vi "Handle Response.vi"(7 "Processing In":refnum<class "Processing.lvclass">, 11 "Response Handler in":refnum<class "Response Handler.lvclass">) -> (0 "error out":errorcluster, 5 "Processing":refnum<class "Processing.lvclass">)   [LabVIEW 2020, in "HTTP Server.lvlib" / "Response Handler.lvclass"]
uses:
  Response Handler.lvclass
  Processing/Processing.lvclass
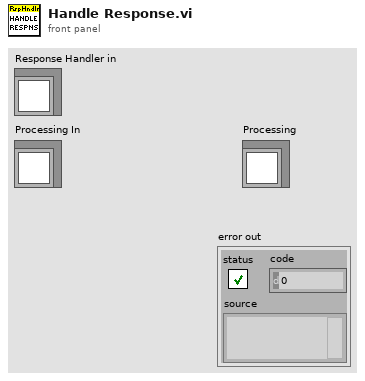
[diagram p1: front panel]
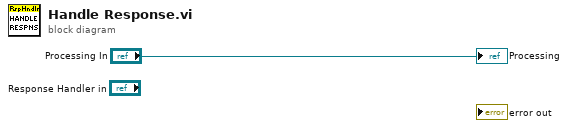
[diagram p0: block diagram]
diagram:
  "Processing" <- "Processing In"
